vi "SETI_FPGA Interface v2.vi"() -> ()   [LabVIEW 2012]
uses:
  <vilib>/rvi/interface/RandomDataEmulation/nirviRandomDataOpen.vi
  <vilib>/rvi/interface/common/niFpgaCacheSessionInfoDynamic.vi
  <vilib>/Utility/error.llb/Error Cluster From Error Code.vi
  <vilib>/rvi/errors/niLvFpgaAdjustHostInterfaceError.vi
  <vilib>/FPGAPlugInAG/Dynamic/niLvFpga_Close_Dynamic.vi
  <vilib>/rvi/interface/nirviOpenFPGA/nirviOpenFPGA.xnode
  SETI_Host_Interface v2.vi
  <vilib>/rvi/interface/nirviReadWriteControl/nirviReadWriteControl.xnode
  <vilib>/rvi/interface/nirviMethod/nirviMethod.xnode
  <vilib>/rvi/interface/nirviCloseFPGA/nirviCloseFPGA.xnode
  <vilib>/rvi/interface/Simulation/niFpgaSimulationCallBeginRW.vi
  <vilib>/rvi/errors/niLvFpgaMergeErrorWithErrorCode.vi
  <vilib>/FPGAPlugInAG/Dynamic/niLvFpga_ReadFifo_Dynamic.vi
  <vilib>/FPGAPlugInAG/Dynamic/niLvFpga_ConfigureFifo_Dynamic.vi
  <vilib>/Analysis/NI_AALBase.lvlib
  NiFpgaLv.dll
  <vilib>/FPGAPlugInAG/Dynamic/niLvFpga_WriteFifo_Dynamic.vi
panel:
  out "%Error":sgl[](array[numeric]) format="%_4e"
  out "Waveform Graph":sgl[][](graph)
  in  "Inputs":i32=2500
  out "Ok?":bool
  out "FPGA Loop Count":i32
  out "State":T1(ring)
  out "Total":u64
  out "Count":u64
  out "Start":bool
  out "Loop Count":i32
  out "Elements Remaining":u32
  out "Output":u64[](array[numeric])
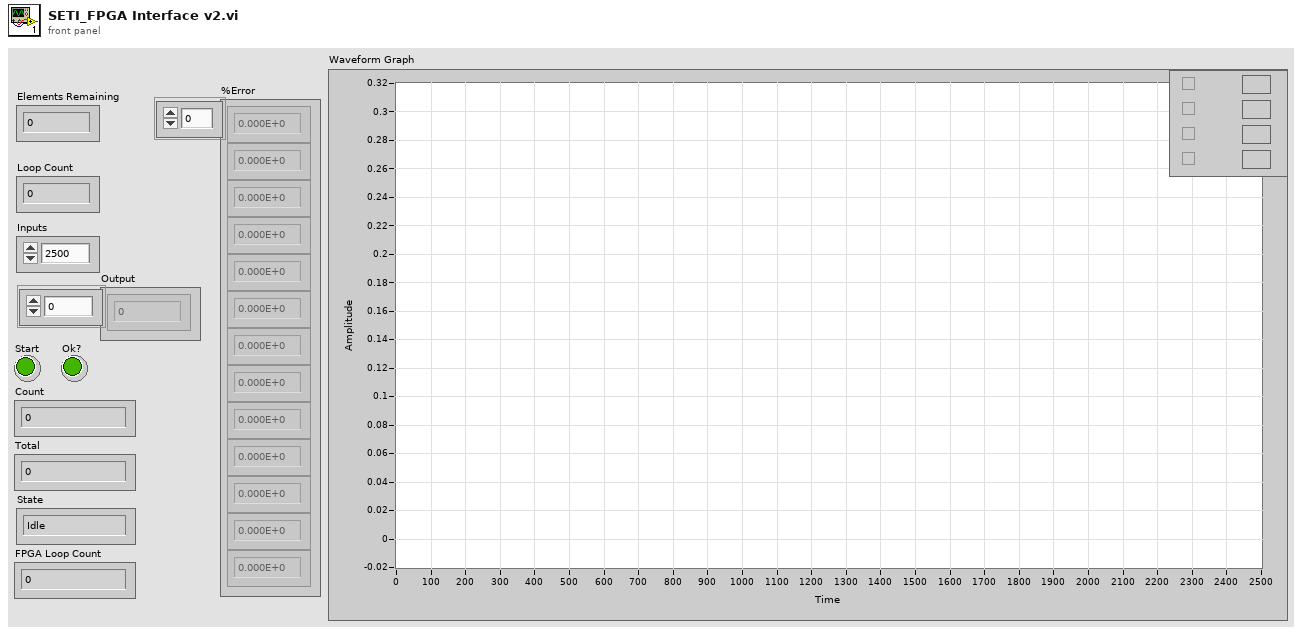
[diagram p1: front panel]
types:
  T1 = enum16{"Idle", "GetNumPoints", "GetChirpRate", "Process", "Stop"}
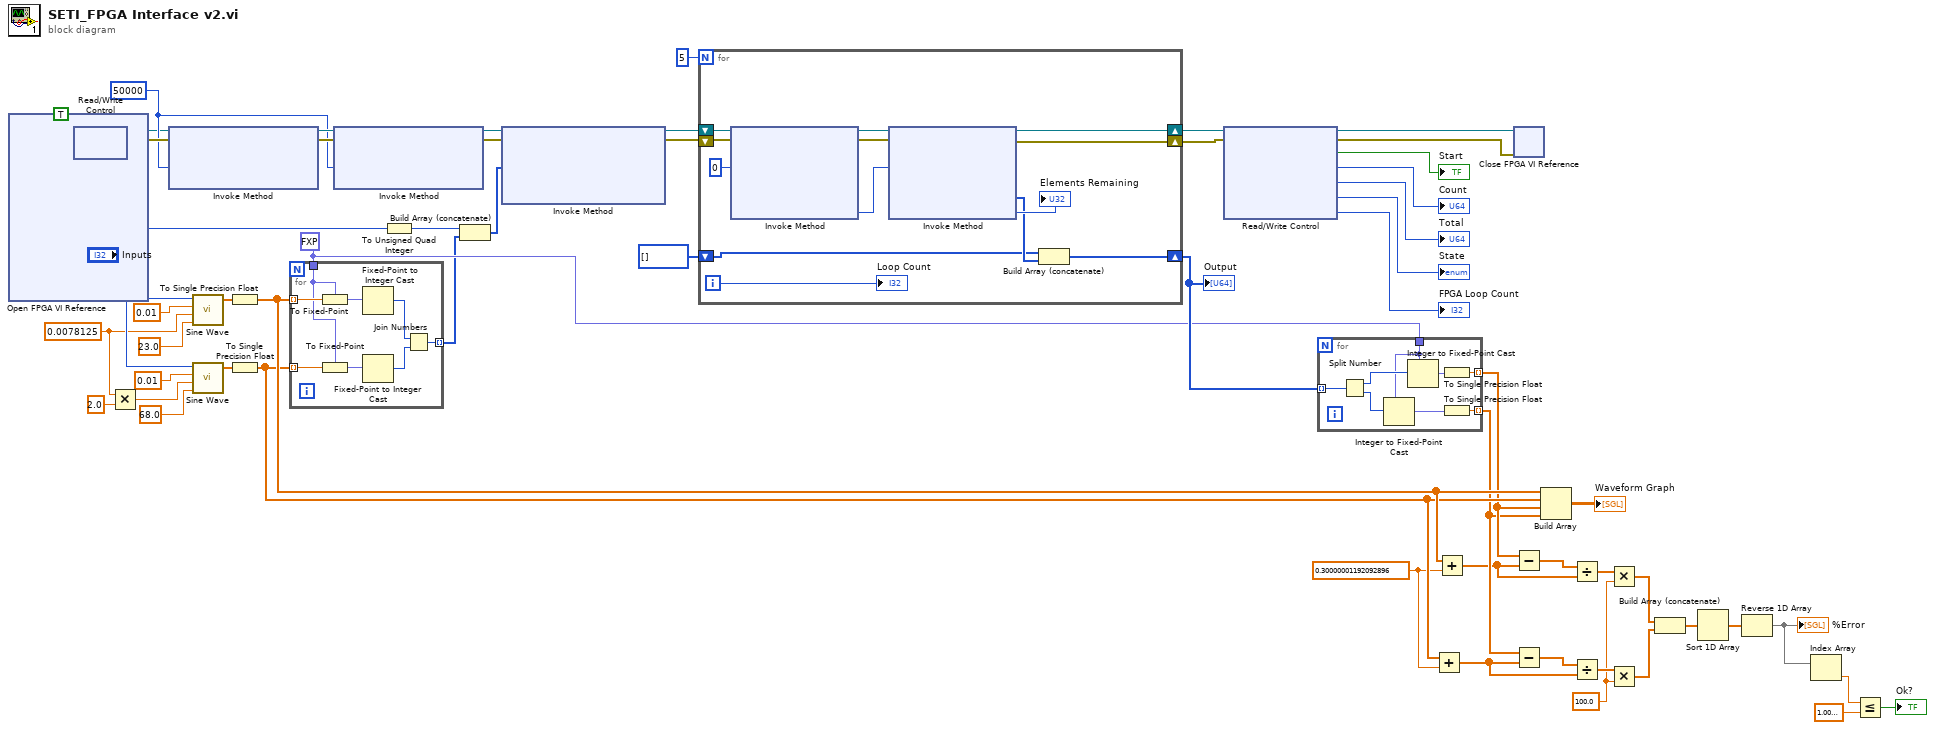
[diagram p0: block diagram]
diagram:
  w10 = sgl 100.0
  w19 = sgl 0.3
  w24 = fxp<+/-,32,1> 0.0 ("real data in")
  w28 = 0.0078125 ("frequency")
  w42 = u32 50000 ("Requested Depth")
  n1 = xnode "Open FPGA VI Reference"() -> ("FPGA VI Reference Out"=w59:refnum<k20>, "error out"=w58:errorcluster)  [unwired: 2 in]
  n2 = xnode "Read/Write Control"("FPGA VI Reference In"=w59, "error in"=w58, "Start"=TRUE ("Boolean")) -> ("FPGA VI Reference Out"=w38:refnum<k20>, "error out"=w45:errorcluster)
  n3 = Multiply(x=w28, y=2.0) -> (x*y=w26:dbl)
  n4 = xnode "Invoke Method"("FPGA VI Reference In"=w38, "error in"=w45, "Requested Depth"=w42) -> ("FPGA VI Reference Out"=w44:refnum<k20>, "error out"=w43:errorcluster)  [unwired: 1 out]
  n5 = call <vilib>:"Sine Wave.vi"("samples"="Inputs", "amplitude"=0.01, "frequency"=w28, "phase in"=23.0) -> ("sine wave"=w31:dbl[])  [unwired: 1 in, 2 out]
  n6 = call <vilib>:"Sine Wave.vi"("samples"="Inputs", "amplitude"=0.01, "frequency"=w26, "phase in"=68.0) -> ("sine wave"=w30:dbl[])  [unwired: 1 in, 2 out]
  n7 = To Single Precision Float(number=w31) -> (single precision float=w21:sgl[])
  n8 = To Single Precision Float(number=w30) -> (single precision float=w20:sgl[])
  n9 = for {
    tunnel: w21 -> [w67] mode=indexing
    tunnel: w20 -> [w63] mode=indexing
    tunnel: [w61] -> w22 mode=indexing
    tunnel: w24 -> [w60]
    n10 = To Fixed-Point(fixed-point type=w60, number=w67) -> (fixed-point=w66:fxp<+/-,32,1>)
    n11 = To Fixed-Point(fixed-point type=w60, number=w63) -> (fixed-point=w64:fxp<+/-,32,1>)
    n12 = Fixed-Point to Integer Cast(1:w66) -> (0:w65:i32)
    n13 = Fixed-Point to Integer Cast(1:w64) -> (0:w62:i32)
    n14 = Join Numbers(hi=w65, lo=w62) -> ((hi.lo)=w61:u64)
  }
  n15 = xnode "Invoke Method"("FPGA VI Reference In"=w44, "error in"=w43, "Requested Depth"=w42) -> ("FPGA VI Reference Out"=w41:refnum<k20>, "error out"=w40:errorcluster)  [unwired: 1 out]
  n16 = To Unsigned Quad Integer(1:"Inputs") -> (0:w36:u64)
  n17 = Build Array (concatenate)(w36, w22) -> (w37:u64[])
  n18 = xnode "Invoke Method"("FPGA VI Reference In"=w41, "error in"=w40, "Data"=w37) -> ("FPGA VI Reference Out"=w56:refnum<k20>, "error out"=w55:errorcluster)  [unwired: 1 in, 1 out]
  n19 = for {
    N: 5 -> [_]
    shift-right: [w68] -> w25
    shift-left: u64[] [] -> [w78]
    shift-right: [w76] -> w52
    shift-left: w56 -> [w74]
    shift-right: [w75] -> w51
    shift-left: w55 -> [w73]
    i -> [w77]
    n20 = xnode "Invoke Method"("FPGA VI Reference In"=w74, "error in"=w73, "Number of Elements"=u32 0) -> ("FPGA VI Reference Out"=w72:refnum<k20>, "error out"=w71:errorcluster, "Elements Remaining"=w69:u32)  [unwired: 1 in, 1 out]
    n21 = xnode "Invoke Method"("FPGA VI Reference In"=w72, "error in"=w71, "Number of Elements"=w69) -> ("FPGA VI Reference Out"=w76:refnum<k20>, "error out"=w75:errorcluster, "Data"=w79:u64[], "Elements Remaining"=→"Elements Remaining":u32)  [unwired: 1 in]
    n22 = Build Array (concatenate)(w78, w79) -> (w68:u64[])
    "Loop Count" <- w77
  }
  "Output" <- w25
  n23 = xnode "Read/Write Control"("FPGA VI Reference In"=w52, "error in"=w51) -> ("FPGA VI Reference Out"=w47:refnum<k20>, "error out"=w46:errorcluster, "Start"=→"Start":bool, "Count"=→"Count":u64, "Total"=→"Total":u64, "State"=→"State":T1, "FPGA Loop Count"=→"FPGA Loop Count":i32)
  n24 = for {
    tunnel: w25 -> [w88] mode=indexing
    tunnel: [w87] -> w18 mode=indexing
    tunnel: [w86] -> w17 mode=indexing
    tunnel: w24 -> [w83]
    n25 = Split Number(x=w88) -> (hi(x)=w85:u32, lo(x)=w84:u32)
    n26 = Integer to Fixed-Point Cast(fixed-point type=w83, integer=w84) -> (fixed-point=w81:fxp<+/-,32,1>)
    n27 = Integer to Fixed-Point Cast(fixed-point type=w83, integer=w85) -> (fixed-point=w82:fxp<+/-,32,1>)
    n28 = To Single Precision Float(number=w82) -> (single precision float=w87:sgl)
    n29 = To Single Precision Float(number=w81) -> (single precision float=w86:sgl)
  }
  n30 = Add(x=w20, y=w19) -> (x+y=w13:sgl[])
  n31 = Add(x=w21, y=w19) -> (x+y=w15:sgl[])
  n32 = xnode "Close FPGA VI Reference"("FPGA VI Reference In"=w47, "error in"=w46) -> ()  [unwired: 1 out]
  n33 = Subtract(x=w18, y=w15) -> (x-y=w16:sgl[])
  n34 = Subtract(x=w17, y=w13) -> (x-y=w14:sgl[])
  n35 = Build Array(w21, w20, w18, w17) -> (→"Waveform Graph":sgl[][])
  n36 = Divide(x=w16, y=w15) -> (x/y=w12:sgl[])
  n37 = Divide(x=w14, y=w13) -> (x/y=w11:sgl[])
  n38 = Multiply(x=w12, y=w10) -> (x*y=w9:sgl[])
  n39 = Multiply(x=w11, y=w10) -> (x*y=w8:sgl[])
  n40 = Build Array (concatenate)(w9, w8) -> (w7:sgl[])
  n41 = Sort 1D Array(array=w7) -> (sorted array=w6:sgl[])
  n42 = Reverse 1D Array(array=w6) -> (reversed array=w5:sgl[])
  "%Error" <- w5
  n43 = Index Array(array=w5) -> (element=w4:sgl)  [unwired: 1 in]
  n44 = Less Or Equal?(x=w4, y=sgl 1e-07) -> (x <= y?=→"Ok?":bool)
